vi "io.main.vi"   [LabVIEW 2019]
uses:
  <vilib>/rvi/eio/common/nirviEmuTemplateMethod_errors.vi
  <vilib>/rvi/Emulation/niFpgaEmulationIsFPGAContextNoSignature.vi
  <vilib>/rvi/DataTransferAndStorage/Container/Common/niFpgaContainerGetUniqueNameForEmu.vi
  <vilib>/rvi/Memory/Memory_Emulation/niFpgaMemoryEmulationCacheClearOnFirstRun.vi
  <vilib>/rvi/Memory/Memory_Emulation/nirvimemoryEmulationManagerCache_MakeExclusive.vi
  <vilib>/rvi/Memory/Memory_Emulation/niFpgaMemoryEmulationValidateCache.vi
  <vilib>/rvi/Memory/Memory_Emulation/nirvimemoryEmulationManagerCache_InsertValue.vi
  <vilib>/Utility/error.llb/Clear Errors.vi
  <vilib>/rvi/Memory/Memory_Emulation/nirvimemoryEmulationManagerCache_ReleaseExclusive.vi
  <vilib>/rvi/Memory/Memory_Emulation/nirvimemoryEmulationManagerCache_GetValue.vi
  <vilib>/rvi/Memory/Memory_Emulation/nirvimemoryEmulationManagerCache_SetValue.vi
  <vilib>/rvi/Emulation/niFpgaProcessEmulError.vi
  <vilib>/rvi/Emulation/niFpgaSctlEmulationGetInTimedLoop.vi
  rti.global.vi
  <vilib>/eio/EIONode/EIONode.xnode
  <vilib>/rvi/DataTransferAndStorage/Container/XNode/niFpgaContainer.xnode
  <vilib>/rvi/DataTransferAndStorage/Register/Emulation/niFpgaRegisterEmulation.vi
types:
  T1 = cluster{"home":fxp<+/-,32,2>, "counts":u64, "reference":u64, "step":u64, "negate?":bool}
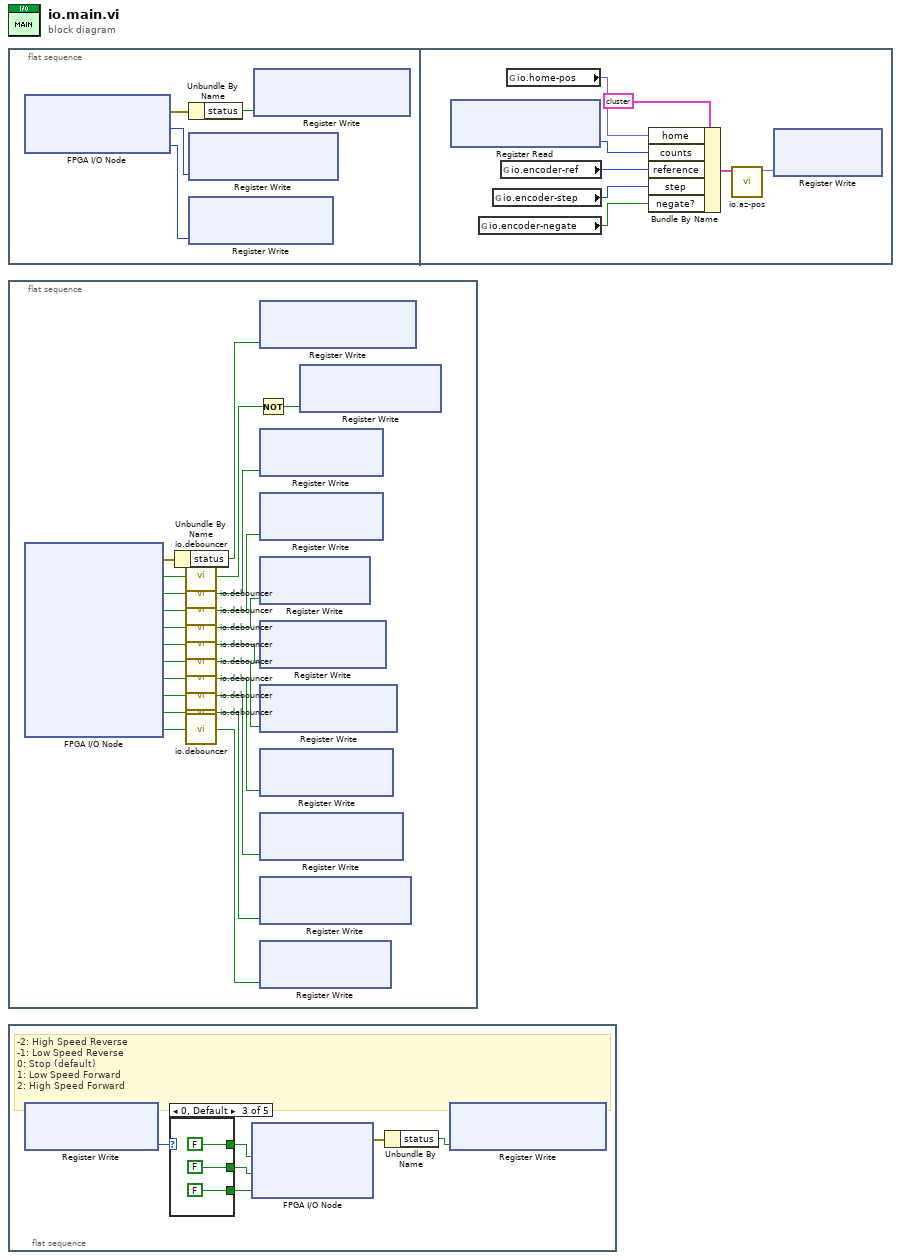
[diagram p0: block diagram]
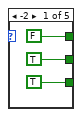
[diagram p2: hidden frame]
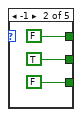
[diagram p3: hidden frame]
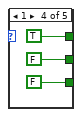
[diagram p4: hidden frame]
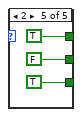
[diagram p5: hidden frame]
diagram:
  n1 = flat-sequence {
    frame #0 {
      n2 = xnode "FPGA I/O Node"() -> ("error out"=w2:errorcluster, "Mod4/Ch1 Abs Pos"=w3:u64, "Mod4/Ch1 Status"=w4:u16)  [unwired: 3 in, 2 out]
      n3 = Unbundle By Name(w2) -> ("status"=w1:bool)
      n4 = xnode "Register Write"("Data"=w3) -> ()  [unwired: 1 in, 1 out]
      n5 = xnode "Register Write"("Data"=w4) -> ()  [unwired: 1 in, 1 out]
      n6 = xnode "Register Write"("Data"=w1) -> ()  [unwired: 1 in, 1 out]
    }
    frame #1 {
      n7 = xnode "Register Read"() -> ("Data"=w7:u64)  [unwired: 1 in, 1 out]
      n8 = global read "rti.global.vi" "io.encoder-negate"() -> (w10:bool)
      n9 = global read "rti.global.vi" "io.encoder-step"() -> (w9:u64)
      n10 = global read "rti.global.vi" "io.encoder-ref"() -> (w8:u64)
      n11 = global read "rti.global.vi" "io.home-pos"() -> (w6:fxp<+/-,32,2>)
      n12 = Bundle By Name(cluster=T1 {"home"=0.0, "counts"=0, "reference"=0, "step"=10000, "negate?"=FALSE}, "home"=w6, "counts"=w7, "reference"=w8, "step"=w9, "negate?"=w10) -> (w5:T1)
      n13 = call "io.az-pos.vi"("Cluster"=w5) -> ("Numeric"=w12:fxp<+/-,32,2>)  [unwired: 10 in]
      n14 = xnode "Register Write"("Data"=w12) -> ()  [unwired: 1 in, 1 out]
    }
  }
  n15 = flat-sequence {
    frame #0 {
      n16 = xnode "FPGA I/O Node"() -> ("error out"=w35:errorcluster, "EM STOP Button"=w33:bool, "CLOSE Button"=w32:bool, "OPEN Button"=w30:bool, "UP Button"=w28:bool, "DOWN Button"=w26:bool, "FORWARD Button"=w24:bool, "REVERSE Button"=w22:bool, "AZ HOME Sensor"=w20:bool, "FORCE STOP"=w14:bool, "ENV Sensor"=w18:bool)  [unwired: 11 in, 10 out]
      n17 = Unbundle By Name(w35) -> ("status"=w34:bool)
      n18 = call "io.debouncer.vi"("input"=w33) -> ("output"=w15:bool)  [unwired: 1 in]
      n19 = call "io.debouncer.vi"("input"=w32) -> ("output"=w31:bool)  [unwired: 1 in]
      n20 = call "io.debouncer.vi"("input"=w30) -> ("output"=w29:bool)  [unwired: 1 in]
      n21 = call "io.debouncer.vi"("input"=w28) -> ("output"=w27:bool)  [unwired: 1 in]
      n22 = call "io.debouncer.vi"("input"=w26) -> ("output"=w25:bool)  [unwired: 1 in]
      n23 = call "io.debouncer.vi"("input"=w24) -> ("output"=w23:bool)  [unwired: 1 in]
      n24 = call "io.debouncer.vi"("input"=w22) -> ("output"=w21:bool)  [unwired: 1 in]
      n25 = call "io.debouncer.vi"("input"=w20) -> ("output"=w19:bool)  [unwired: 1 in]
      n26 = call "io.debouncer.vi"("input"=w14) -> ("output"=w13:bool)  [unwired: 1 in]
      n27 = call "io.debouncer.vi"("input"=w18) -> ("output"=w17:bool)  [unwired: 1 in]
      n28 = Not(x=w15) -> (.not. x?=w16:bool)
      n29 = xnode "Register Write"("Data"=w34) -> ()  [unwired: 1 in, 1 out]
      n30 = xnode "Register Write"("Data"=w31) -> ()  [unwired: 1 in, 1 out]
      n31 = xnode "Register Write"("Data"=w29) -> ()  [unwired: 1 in, 1 out]
      n32 = xnode "Register Write"("Data"=w27) -> ()  [unwired: 1 in, 1 out]
      n33 = xnode "Register Write"("Data"=w25) -> ()  [unwired: 1 in, 1 out]
      n34 = xnode "Register Write"("Data"=w23) -> ()  [unwired: 1 in, 1 out]
      n35 = xnode "Register Write"("Data"=w21) -> ()  [unwired: 1 in, 1 out]
      n36 = xnode "Register Write"("Data"=w19) -> ()  [unwired: 1 in, 1 out]
      n37 = xnode "Register Write"("Data"=w13) -> ()  [unwired: 1 in, 1 out]
      n38 = xnode "Register Write"("Data"=w17) -> ()  [unwired: 1 in, 1 out]
      n39 = xnode "Register Write"("Data"=w16) -> ()  [unwired: 1 in, 1 out]
    }
  }
  n40 = flat-sequence {
    frame #0 {
      # "-2: High Speed Reverse\n-1: Low Speed Reverse\n0: Stop (default)\n1: Low Speed Forward\n2: High Speed Forward"
      n41 = xnode "Register Write"() -> ("Data"=w41:i8)  [unwired: 1 in, 1 out]
      n42 = case shown="0, Default" w41 {
        tunnel: [FALSE ("Forward Dome") FALSE ("Forward Dome") FALSE ("Forward Dome") TRUE ("Forward Dome") TRUE ("Forward Dome")] -> w40
        tunnel: [TRUE ("Reverse Dome") TRUE ("Reverse Dome") FALSE ("Reverse Dome") FALSE ("Reverse Dome") FALSE ("Reverse Dome")] -> w39
        tunnel: [TRUE ("High Speed") FALSE ("High Speed") FALSE ("High Speed") FALSE ("High Speed") TRUE ("High Speed")] -> w38
        frame -2 {
        }
        frame -1 {
        }
        frame 0, Default {
        }
        frame 1 {
        }
        frame 2 {
        }
      }
      n43 = xnode "FPGA I/O Node"("Forward Dome"=w40, "Reverse Dome"=w39, "High Speed"=w38) -> ("error out"=w37:errorcluster)  [unwired: 4 in, 3 out]
      n44 = Unbundle By Name(w37) -> ("status"=w36:bool)
      n45 = xnode "Register Write"("Data"=w36) -> ()  [unwired: 1 in, 1 out]
    }
  }
